vi "Main.vi"(11 "Module Admin":refnum<class "Delacor_lib_QMH_Module Admin.lvclass">) -> ()   [LabVIEW 2019, in "FunctionGenerator.lvlib"]
doc: "This template is based off of the Queued Message Handler design pattern and the Queued Message Handler project template that ships with LabVIEW.\n\nThe main difference is that the queue is private to this module and communication between modules is performed via Broadcast and Request events.\n\nRequest events are wrapped in public API methods and are handled in the Event Handling Loop (EHL) of this VI. Any module can register for Broadcast events sent by this module. The EHL generates messages based on user interface actions.\n\nThe Message Handling Loop (MHL) processes messages generated by the EHL, or by other messages. The messages are string values, so new messages can be added easily to the Message Cases case structure in the MHL. Each message cluster can also provide an optional value for Message Data, which is a variant that can be converted to whatever message-specific data is required.\n_____\nBased on DQMH Dev Tools: Project Template 7.1.0.1503."
uses:
  FunctionGenerator.lvlib
  <vilib>/Delacor/Delacor QMH/Libraries/Module Admin_class/Delacor_lib_QMH_Module Admin.lvclass
  Module Data--cluster.ctl
  Wake UP Continuous HL Argument--cluster.ctl
  <vilib>/Delacor/Delacor QMH/Libraries/Message Queue_class/Delacor_lib_QMH_Message Queue.lvclass/Delacor_lib_QMH_Message Queue.ctl
  Stop Argument--cluster.ctl
  <vilib>/Delacor/Delacor QMH/Libraries/Module Admin_class/Delacor_lib_QMH_Module Admin.lvclass/Delacor_lib_QMH_Module Admin.ctl
  Set Amplitude Argument--cluster.ctl
  Set Offset Argument--cluster.ctl
  Set Frecuency Argument--cluster.ctl
  Set Signal Type Argument--cluster.ctl
  Get Waveform Argument--cluster.ctl
  Get Waveform (Reply Payload)--cluster.ctl
  Start Continuous Acquisition Argument--cluster.ctl
  <vilib>/Utility/miscctls.llb/LVPointTypeDef.ctl
  <vilib>/Delacor/Delacor QMH/Libraries/Message Queue_class/Delacor_lib_QMH_Enqueue Message (Single).vi
  <vilib>/Delacor/Delacor QMH/Libraries/Module Admin_class/Delacor_lib_QMH_Get External Launch.vi
  <vilib>/Delacor/Delacor QMH/Libraries/Message Queue_class/Delacor_lib_QMH_Message Queue.lvclass
  <vilib>/measure/NI_MABase.lvlib
panel:
  out "error out":errorcluster
  out "Status":string
  in  "Simulate MHL Error":bool
  in  "Simulate EHL Error":bool
  # "Other processes communicate with this Module via its Public API (wrappers for its Request Events).\n\nThis Module communicates with other processes via its Broadcast Events.\nAny process that wants to receive these messages can register for this module's Broadcast events."
  # "This template is for the DQMH framework. See the block diagram for more information on how to use this template."
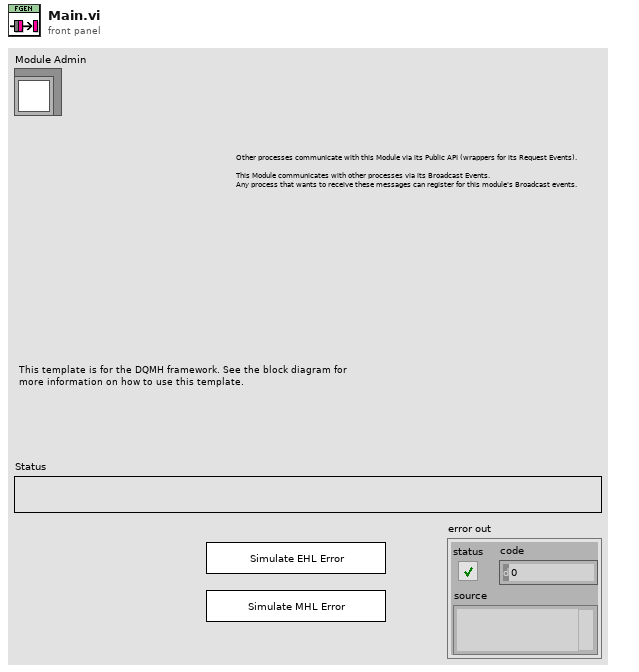
[diagram p1: front panel]
types:
  T1 = typedef "FunctionGenerator.lvlib/Request Events--cluster.ctl" = cluster{"Stop Module":refnum<user-event>, "Show Panel":refnum<user-event>, "Hide Panel":refnum<user-event>, "Get Module Execution Status":refnum<user-event>, "Show Diagram":refnum<user-event>, "Set Amplitude":refnum<user-event>, "Set Offset":refnum<user-event>, "Set Frecuency":refnum<user-event>, "Set Signal Type":refnum<user-event>, "Get Waveform":refnum<user-event>, "Private.Wake UP Continuous HL":refnum<user-event>, "Start Continuous Acquisition":refnum<user-event>, "Stop Continuous Generation":refnum<user-event>}
  T2 = typedef "FunctionGenerator.lvlib/Module Data--cluster.ctl" = cluster{"Status":string, "Amplitude":dbl, "Frecuency":dbl, "Offset":dbl, "signal type":enum16{"Sine Wave", "Triangle Wave", "Square Wave", "Sawtooth Wave"}}
  T3 = typedef "FunctionGenerator.lvlib/Wake UP Continuous HL Argument--cluster.ctl" = cluster{"Amplitude":dbl, "Frecuency":dbl, "Offset":dbl, "signal type":enum16{"Sine Wave", "Triangle Wave", "Square Wave", "Sawtooth Wave"}}
  T4 = enum32{"invalid lock state", "Not Locked", "Locked (No Password)", "Password-protected"}
  T5 = typedef "FunctionGenerator.lvlib/Stop Argument--cluster.ctl" = cluster{"Origin":string, "Exit via Stop Module Req?":bool, "Wait for Module to stop?":bool}
  T6 = typedef "FunctionGenerator.lvlib/Set Amplitude Argument--cluster.ctl" = cluster{"Amplitude":dbl}
  T7 = typedef "FunctionGenerator.lvlib/Set Offset Argument--cluster.ctl" = cluster{"Offset":dbl}
  T8 = typedef "FunctionGenerator.lvlib/Set Frecuency Argument--cluster.ctl" = cluster{"Frecuency":dbl}
  T9 = typedef "FunctionGenerator.lvlib/Set Signal Type Argument--cluster.ctl" = cluster{"signal type":enum16{"Sine Wave", "Triangle Wave", "Square Wave", "Sawtooth Wave"}}
  T10 = typedef "FunctionGenerator.lvlib/Get Waveform Argument--cluster.ctl" = cluster{"Wait Notifier":refnum<notifier>, "wait for reply":bool}
  T11 = typedef "FunctionGenerator.lvlib/Start Continuous Acquisition Argument--cluster.ctl" = cluster{"Boolean":bool}
  T12 = typedef "LVPointTypeDef.ctl" = cluster{"Horizontal":i16, "Vertical":i16}
  T13 = enum32{"Invalid", "Standard", "Closed", "Hidden", "Minimized", "Maximized"}
  T14 = typedef "FunctionGenerator.lvlib/Get Waveform (Reply Payload)--cluster.ctl" = cluster{"Waveform":waveform(dbl), "error":errorcluster}
  T15 = enum16{"Sine Wave", "Triangle Wave", "Square Wave", "Sawtooth Wave"}
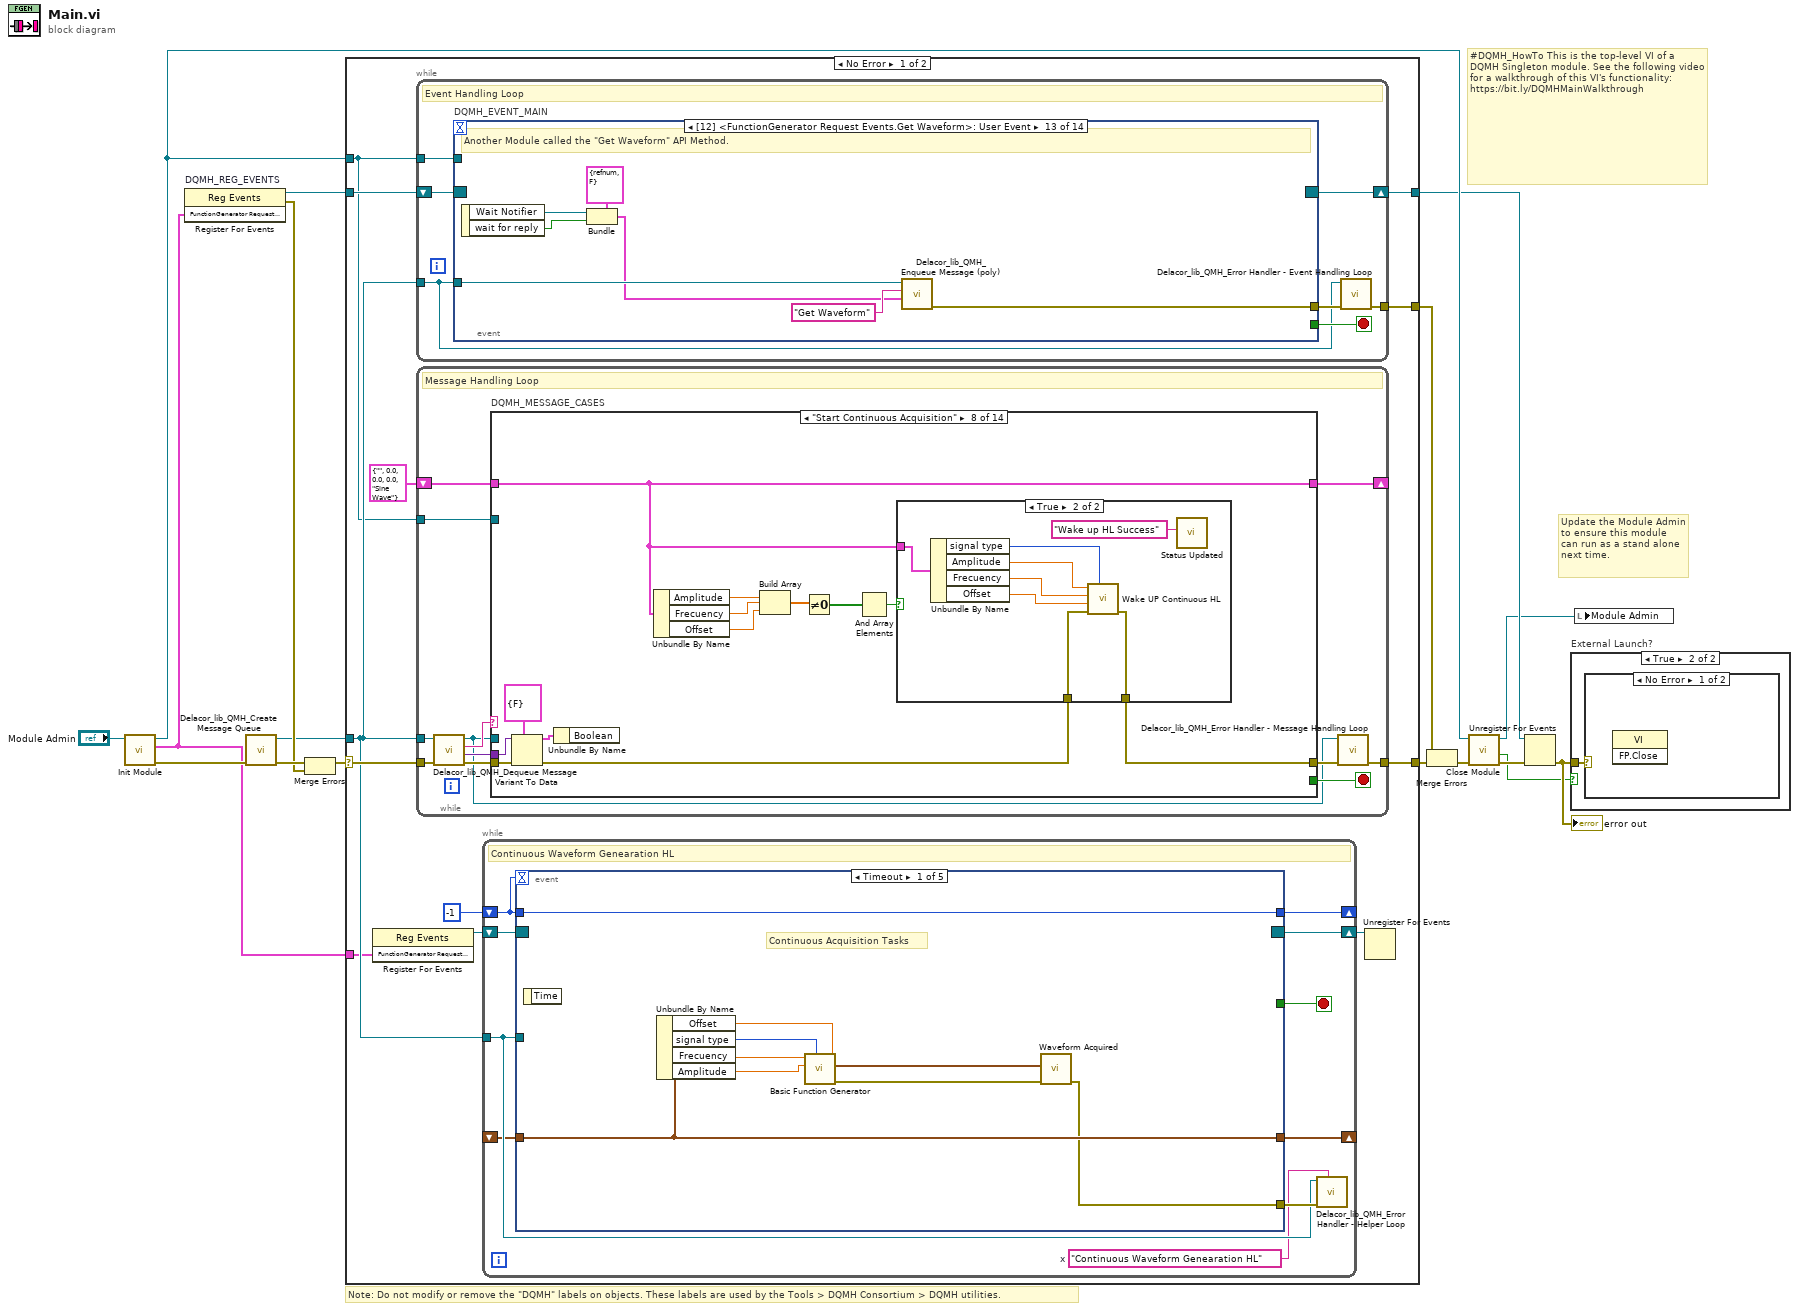
[diagram p0: block diagram]
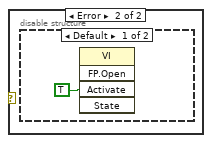
[diagram p3: hidden frame]
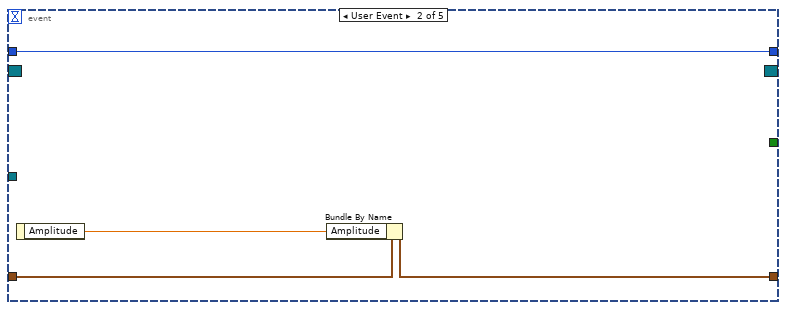
[diagram p5: hidden frame]
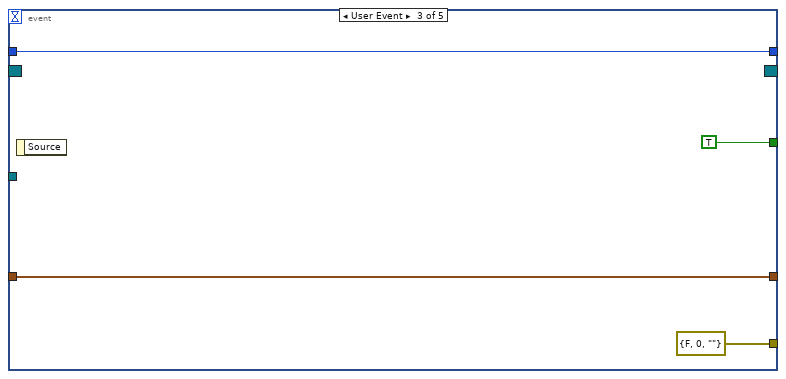
[diagram p6: hidden frame]
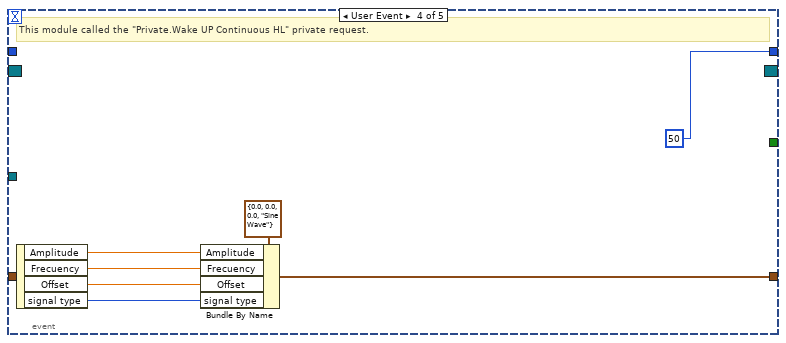
[diagram p7: hidden frame]
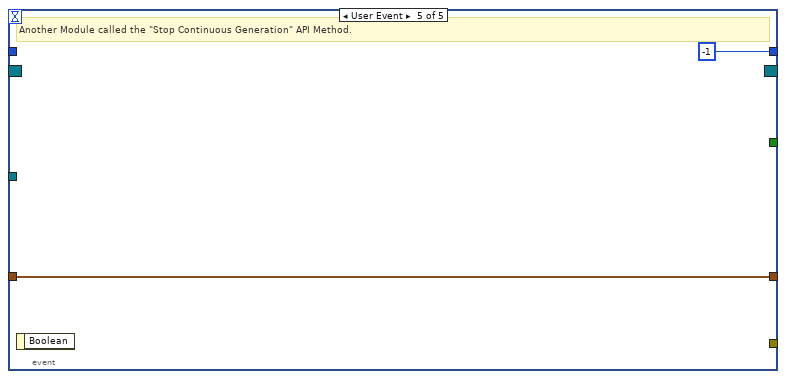
[diagram p8: hidden frame]
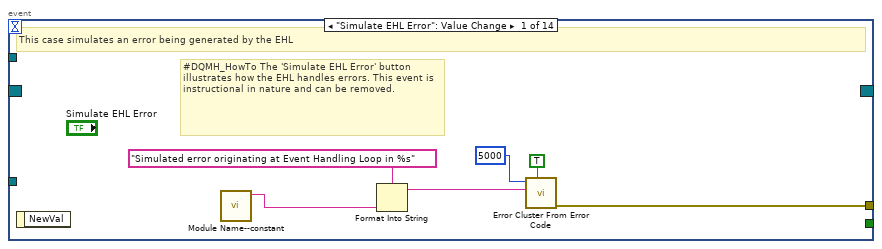
[diagram p9: hidden frame]
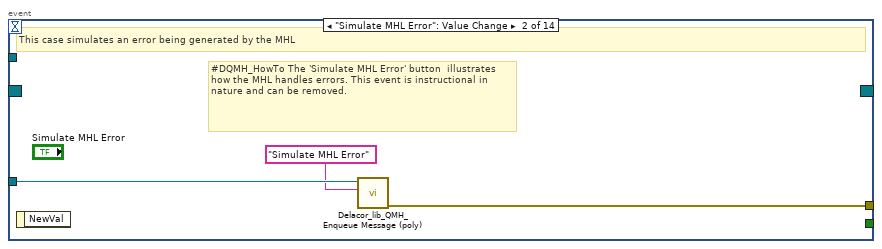
[diagram p10: hidden frame]
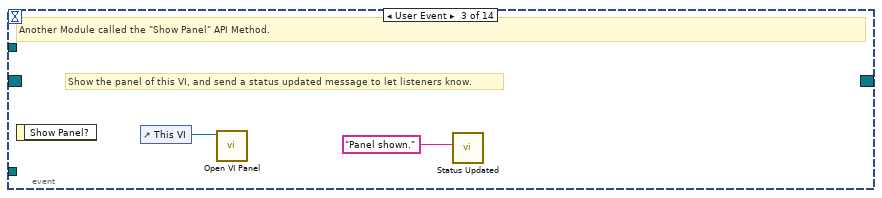
[diagram p11: hidden frame]
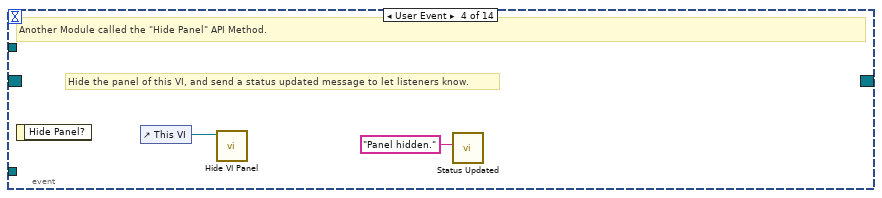
[diagram p12: hidden frame]
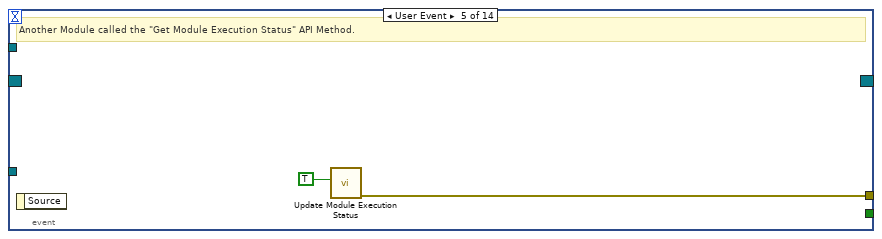
[diagram p13: hidden frame]
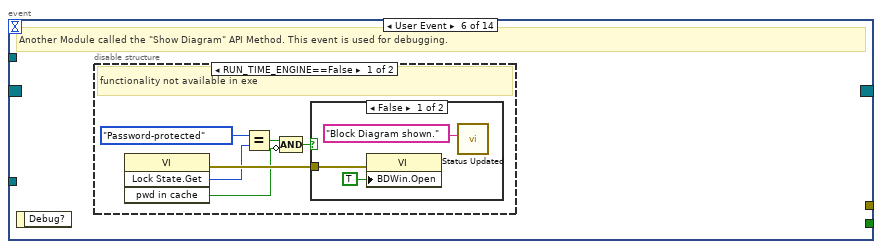
[diagram p14: hidden frame]
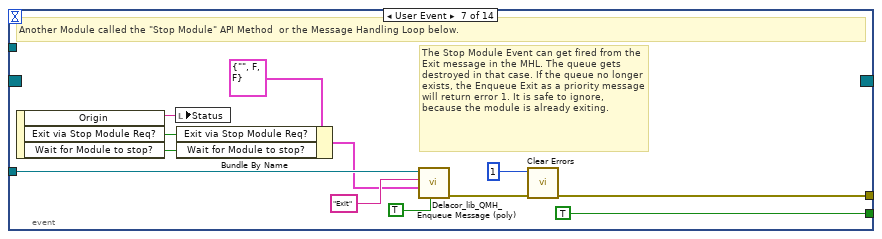
[diagram p17: hidden frame]
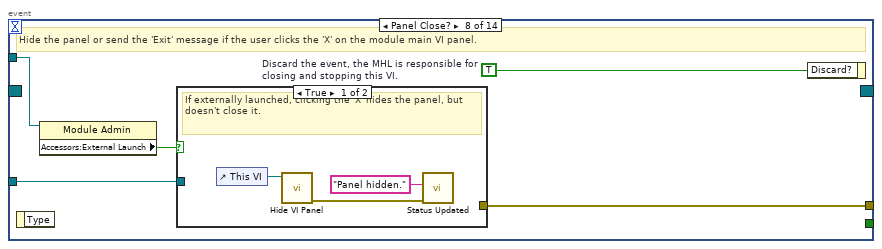
[diagram p18: hidden frame]
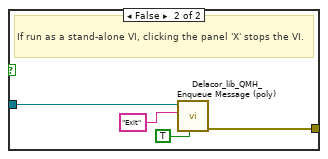
[diagram p19: hidden frame]
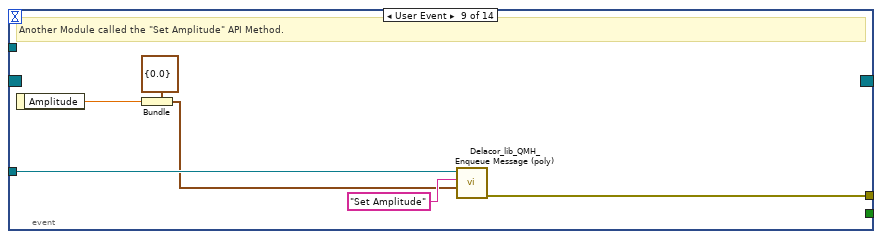
[diagram p20: hidden frame]
diagram:
  # "#DQMH_HowTo This is the top-level VI of a DQMH Singleton module. See the following video for a walkthrough of this VI's functionality: https://bit.ly/DQMHMainWalkthrough"
  # "Note: Do not modify or remove the \"DQMH\" labels on objects. These labels are used by the Tools > DQMH Consortium > DQMH utilities."
  # "Update the Module Admin to ensure this module can run as a stand alone next time."
  n1 = call "Init Module.vi"("Singleton Module Admin in"="Module Admin") -> ("error out"=w16:errorcluster, "FunctionGenerator Request Events"=w1:T1, "Singleton Module Admin out"=w8:refnum<class "Delacor_lib_QMH_Module Admin.lvclass">)  [unwired: 8 in]
  n2 = register-events "DQMH_REG_EVENTS"(w1) -> (reference out=w6:refnum<event-registration>, error out=w9:errorcluster)  [unwired: 2 in]
  n3 = call <vilib>:"Delacor_lib_QMH_Create Message Queue.vi"("error in"=w16) -> ("error out"=w11:errorcluster, "Message Queue"=w5:refnum<class "Delacor_lib_QMH_Message Queue.lvclass">)  [unwired: 9 in]
  n4 = Merge Errors(w11, w9) -> (w10:errorcluster)
  n5 = case shown="No Error" w10 {
    selector: w10 -> [w27 w336]
    tunnel: [w29 w335] -> w17
    tunnel: [w26 w334] -> w7
    tunnel: w6 -> [w24 w334]
    tunnel: w5 -> [w23 w329]
    tunnel: [w28 _] -> w14
    tunnel: w8 -> [w22 w330]
    tunnel: w1 -> [w21 _]
    frame No Error {
      n6 = register-events ("DQMH_HELPER_REGFOREVENTS")(w21) -> (reference out=w19:refnum<event-registration>)  [unwired: 2 in, 1 out]
      n7 = while {
        tunnel: w23 -> [w66]
        shift-right: [w69] -> w26
        shift-left: w24 -> [w70]
        tunnel: [w71] -> w28
        tunnel: w22 -> [w67]
        stop <- w68 stop-if-true
        # "Event Handling Loop"
        n8 = event "DQMH_EVENT_MAIN" shown="[12] <FunctionGenerator Request Events.Get Waveform>: User Event" {
          selector: w70 -> [_ _ _ _ _ _ _ _ _ _ _ _ _ _]
          dyn-events: [_ _ _ _ _ _ _ _ _ _ _ _ _ _] -> w69
          timeout: _ -> [_ _ _ _ _ _ _ _ _ _ _ _ _ _]
          tunnel: [_ _ _ _ _ _ TRUE ("Discard?") _ _ _ _ _ _ _] -> w68
          tunnel: w66 -> [_ w80 _ _ _ _ w104 w111 w125 w131 w137 w144 w151 w157]
          tunnel: [w78 w81 _ _ w87 _ w107 w113 w126 w132 w138 w139 w145 w152] -> w72
          tunnel: w67 -> [_ _ _ _ _ _ _ w110 _ _ _ _ _ _]
          event "Simulate EHL Error": Value Change {
            # "#DQMH_HowTo The 'Simulate EHL Error' button  illustrates how the EHL handles errors. This event is instructional in nature and can be removed."
            # "This case simulates an error being generated by the EHL"
            n9 = event-data() -> ()  [unwired: 1 in, 1 out]
            n10 = call "Module Name--constant.vi"() -> ("Module Name"=w75:string)  [unwired: 11 in]
            n11 = Format Into String(format string="Simulated error originating at Event Handling Loop in %s", w75) -> (resulting string=w76:string)  [unwired: 2 in, 1 out]
            n12 = call <vilib>:"Error Cluster From Error Code.vi"("show call chain? (False)"=TRUE, "error message (\"\")"=w76, "error code (0)"=5000) -> ("error out"=w78:errorcluster)  [unwired: 6 in]
          }
          event "Simulate MHL Error": Value Change {
            # "#DQMH_HowTo The 'Simulate MHL Error' button  illustrates how the MHL handles errors. This event is instructional in nature and can be removed."
            # "This case simulates an error being generated by the MHL"
            n13 = event-data() -> ()  [unwired: 1 in, 1 out]
            n14 = call-poly <vilib>:"Delacor_lib_QMH_Enqueue Message (poly).vi"("Message"="Simulate MHL Error", "Message Queue in"=w80) -> ("error out"=w81:errorcluster)  [unwired: 8 in, 1 out]
          }
          event User Event {
            # "Show the panel of this VI, and send a status updated message to let listeners know."
            # "Another Module called the \"Show Panel\" API Method."
            n15 = event-data() -> ()  [unwired: 1 in, 1 out]
            n16 = control-ref of="This VI"() -> (w83:refnum<vi>)
            n17 = call "Open VI Panel.vi"("VI"=w83) -> ()  [unwired: 10 in, 1 out]
            n18 = call "Status Updated.vi"("Status"="Panel shown." ("format string")) -> ()  [unwired: 10 in, 1 out]
          }
          event User Event {
            # "Hide the panel of this VI, and send a status updated message to let listeners know."
            # "Another Module called the \"Hide Panel\" API Method."
            n19 = event-data() -> ()  [unwired: 1 in, 1 out]
            n20 = control-ref of="This VI"() -> (w85:refnum<vi>)
            n21 = call "Hide VI Panel.vi"("VI"=w85) -> ()  [unwired: 10 in, 1 out]
            n22 = call "Status Updated.vi"("Status"="Panel hidden." ("format string")) -> ()  [unwired: 10 in, 1 out]
          }
          event User Event {
            # "Another Module called the \"Get Module Execution Status\" API Method."
            n23 = event-data() -> ()  [unwired: 1 in, 1 out]
            n24 = call "Update Module Execution Status.vi"("Running?"=TRUE) -> ("error out"=w87:errorcluster)  [unwired: 10 in]
          }
          event User Event {
            # "Another Module called the \"Show Diagram\" API Method. This event is used for debugging."
            n25 = event-data() -> ()  [unwired: 1 in, 1 out]
            n26 = disable-structure shown="RUN_TIME_ENGINE==False" {
              frame condition #0 (active) {
                # "functionality not available in exe"
                n27 = invoke on="Invoke Node" class="VI" method="Lock State.Get"() -> (error out=w93:errorcluster, "Get Lock State"=w92:T4, "pwd in cache"=w89:bool)  [unwired: 4 in, 1 out]
                n28 = Equal?(x=T4."Password-protected", y=w92) -> (x = y?=w90:bool)
                n29 = Compound Arithmetic op=AND(w90, invert w89) -> (w88:bool)
                n30 = case shown="False" w88 {
                  tunnel: w93 -> [w96 _]
                  frame False {
                    n31 = property on="Property Node" class="VI"(error in=w96, "BDWin.Open"=TRUE ("Block Diagram Window:Open")) -> ()  [unwired: 1 in, 2 out]
                    n32 = call "Status Updated.vi"("Status"="Block Diagram shown." ("format string")) -> ()  [unwired: 10 in, 1 out]
                  }
                  frame True {
                    # "Password-protected VI, and the password is not in the cache. Do not show the diagram."
                  }
                }
              }
              frame condition #1 {
              }
            }
          }
          event User Event {
            # "The Stop Module Event can get fired from the Exit message in the MHL. The queue gets destroyed in that case. If the queue no longer exists, the Enqueue Exit as a priority message will return error 1. It is safe to ignore, because the module is already exiting."
            # "Another Module called the \"Stop Module\" API Method  or the Message Handling Loop below."
            n33 = event-data() -> ("Origin"=w103:string, "Exit via Stop Module Req?"=w99:bool, "Wait for Module to stop?"=w98:bool)  [unwired: 1 in]
            n34 = local write "Status"(w103) -> ()
            n35 = Bundle By Name(cluster=T5 {"Origin"="", "Exit via Stop Module Req?"=FALSE, "Wait for Module to stop?"=FALSE} ("Stop Argument"), "Exit via Stop Module Req?"=w99, "Wait for Module to stop?"=w98) -> (w97:T5)
            n36 = call-poly <vilib>:"Delacor_lib_QMH_Enqueue Message (poly).vi"("Priority Message? (F)"=TRUE, "Message Data"=w97, "Message"="Exit", "Message Queue in"=w104) -> ("error out"=w108:errorcluster)  [unwired: 6 in, 1 out]
            n37 = call <vilib>:"Clear Errors.vi"("error in (no error)"=w108, "specific error code to clear (0: all)"=1) -> ("error out"=w107:errorcluster)  [unwired: 4 in, 1 out]
          }
          event Panel Close? {
            w112 = TRUE  # Discard the event, the MHL is responsible for closing and stopping this VI.
            # "Hide the panel or send the 'Exit' message if the user clicks the 'X' on the module main VI panel."
            n38 = event-data() -> ()  [unwired: 1 in, 1 out]
            n39 = property on="Property Node" class="Module Admin"(reference=w110) -> ("Accessors:External Launch"=w109:bool)  [unwired: 1 in, 2 out]
            n40 = case shown="True" w109 {
              tunnel: w111 -> [_ w119]
              tunnel: [_ w120] -> w113
              frame True {
                # "If externally launched, clicking the 'X' hides the panel, but doesn't close it."
                n41 = control-ref of="This VI"() -> (w115:refnum<vi>)
                n42 = call "Hide VI Panel.vi"("VI"=w115) -> ("error out"=w116:errorcluster)  [unwired: 10 in]
                n43 = call "Status Updated.vi"("error in"=w116, "Status"="Panel hidden." ("format string")) -> ()  [unwired: 9 in, 1 out]
              }
              frame False {
                # "If run as a stand-alone VI, clicking the panel 'X' stops the VI."
                n44 = call-poly <vilib>:"Delacor_lib_QMH_Enqueue Message (poly).vi"("Priority Message? (F)"=TRUE, "Message"="Exit", "Message Queue in"=w119) -> ("error out"=w120:errorcluster)  [unwired: 7 in, 1 out]
              }
            }
            n45 = event-data ("Event Filter Node")("Discard?"=w112) -> ()  [unwired: 1 in, 1 out]
          }
          event User Event {
            # "Another Module called the \"Set Amplitude\" API Method."
            n46 = event-data() -> ("Amplitude"=w121:dbl)  [unwired: 1 in]
            n47 = Bundle(cluster=T6 {"Amplitude"=0.0} ("Set Amplitude Argument"), "Amplitude"=w121) -> (w122:T6)
            n48 = call-poly <vilib>:"Delacor_lib_QMH_Enqueue Message (poly).vi"("Message Data"=w122, "Message"="Set Amplitude", "Message Queue in"=w125) -> ("error out"=w126:errorcluster)  [unwired: 7 in, 1 out]
          }
          event User Event {
            # "Another Module called the \"Set Offset\" API Method."
            n49 = event-data() -> ("Offset"=w127:dbl)  [unwired: 1 in]
            n50 = Bundle(cluster=T7 {"Offset"=0.0} ("Set Offset Argument"), "Offset"=w127) -> (w128:T7)
            n51 = call-poly <vilib>:"Delacor_lib_QMH_Enqueue Message (poly).vi"("Message Data"=w128, "Message"="Set Offset", "Message Queue in"=w131) -> ("error out"=w132:errorcluster)  [unwired: 7 in, 1 out]
          }
          event User Event {
            # "Another Module called the \"Set Frecuency\" API Method."
            n52 = event-data() -> ("Frecuency"=w133:dbl)  [unwired: 1 in]
            n53 = Bundle(cluster=T8 {"Frecuency"=0.0} ("Set Frecuency Argument"), "Frecuency"=w133) -> (w134:T8)
            n54 = call-poly <vilib>:"Delacor_lib_QMH_Enqueue Message (poly).vi"("Message Data"=w134, "Message"="Set Frecuency", "Message Queue in"=w137) -> ("error out"=w138:errorcluster)  [unwired: 7 in, 1 out]
          }
          event User Event {
            # "Another Module called the \"Set Signal Type\" API Method."
            n55 = event-data() -> ("signal type"=w140:T15)  [unwired: 1 in]
            n56 = Bundle(cluster=T9 {"signal type"=enum."Sine Wave"} ("Set Signal Type Argument"), "signal type"=w140) -> (w141:T9)
            n57 = call-poly <vilib>:"Delacor_lib_QMH_Enqueue Message (poly).vi"("Message Data"=w141, "Message"="Set Signal Type", "Message Queue in"=w144) -> ("error out"=w139:errorcluster)  [unwired: 7 in, 1 out]
          }
          event User Event {
            # "Another Module called the \"Get Waveform\" API Method."
            n58 = event-data() -> ("Wait Notifier"=w147:refnum<notifier>, "wait for reply"=w146:bool)  [unwired: 1 in]
            n59 = Bundle(cluster=T10 {"Wait Notifier"=refnum, "wait for reply"=FALSE} ("Get Waveform Argument"), "Wait Notifier"=w147, "wait for reply"=w146) -> (w148:T10)
            n60 = call-poly <vilib>:"Delacor_lib_QMH_Enqueue Message (poly).vi"("Message Data"=w148, "Message"="Get Waveform", "Message Queue in"=w151) -> ("error out"=w145:errorcluster)  [unwired: 7 in, 1 out]
          }
          event User Event {
            # "Another Module called the \"Start Continuous Acquisition\" API Method."
            n61 = event-data() -> ("Boolean"=w153:bool)  [unwired: 1 in]
            n62 = Bundle(cluster=T11 {"Boolean"=FALSE} ("Start Continuous Acquisition Argument"), "Boolean"=w153) -> (w154:T11)
            n63 = call-poly <vilib>:"Delacor_lib_QMH_Enqueue Message (poly).vi"("Message Data"=w154, "Message"="Start Continuous Acquisition", "Message Queue in"=w157) -> ("error out"=w152:errorcluster)  [unwired: 7 in, 1 out]
          }
        }
        n64 = call-dynamic "Delacor_lib_QMH_Error Handler - Event Handling Loop.vi"("error in"=w72, "Message Queue in"=w66) -> ("dup error in"=w71:errorcluster)  [unwired: 8 in, 1 out]
      }
      n65 = while {
        tunnel: w23 -> [w158]
        shift-right: [w164] -> _
        shift-left: T2 {"Status"="", "Amplitude"=0.0, "Frecuency"=0.0, "Offset"=0.0, "signal type"=enum."Sine Wave"} ("Data Cluster") -> [w165]
        tunnel: w27 -> [w169]
        tunnel: [w167] -> w29
        tunnel: w22 -> [w160]
        stop <- w163 stop-if-true
        # "Message Handling Loop"
        n66 = call-dynamic "Delacor_lib_QMH_Dequeue Message.vi"("error in"=w169, "Message Queue in"=w158) -> ("error out"=w168:errorcluster, "Message Data"=w161:variant, "Message"=w162:string, "Message Queue out"=w159:refnum<class "Delacor_lib_QMH_Message Queue.lvclass">)  [unwired: 6 in]
        n67 = case "DQMH_MESSAGE_CASES" shown="\"Start Continuous Acquisition\"" w162 {
          selector: w162 -> [_ _ _ _ _ _ _ _ _ _ _ _ _ w324]
          tunnel: w159 -> [_ _ _ _ _ _ _ _ _ _ _ w289 w312 _]
          tunnel: w168 -> [w187 w191 w201 w211 w221 w231 w248 w263 w275 w277 w286 w297 w318 w327]
          tunnel: [w185 w191 w200 w210 w220 w229 w239 w258 w274 w277 w285 w293 w313 w328] -> w166
          tunnel: w165 -> [w176 w190 w199 w209 w219 w230 w238 w251 w273 w276 w283 w291 w311 w325]
          tunnel: [w175 w190 w195 w205 w215 w225 w238 w251 w273 w276 w283 w291 w311 w325] -> w164
          tunnel: [_ _ _ _ _ _ _ _ _ _ _ _ w310 _] -> w163
          tunnel: w161 -> [_ _ w198 w208 w218 w228 w246 w262 _ _ _ w290 w309 _]
          tunnel: w160 -> [w177 _ _ _ _ _ _ _ _ _ _ w288 w304 _]
          frame "Initialize" {
            w171 = "Initial Message" ("Initial Message")
            # "#DQMH_CodeNeeded - Initialize the appearance of the front panel."
            # "#DQMH_CodeNeeded - Initialize your state data here."
            # "Initialize - Any operation that needs to be done before the module can receive messages. Synchronize Caller Events.vi will inform Start Module.vi that the module has launched and is ready to receive messages. Module Did Init.vi will broadcast that the module initialized."
            n68 = call "Synchronize Caller Events.vi"("error in"=w187, "Singleton Module Admin in"=w177) -> ("error out"=w186:errorcluster, "Singleton Module Admin out"=w172:refnum<class "Delacor_lib_QMH_Module Admin.lvclass">)  [unwired: 8 in]
            n69 = property on="Property Node" class="Module Admin"(reference=w172) -> ("Accessors:External Launch"=w181:bool)  [unwired: 1 in, 2 out]
            n70 = Select(t=T13."Hidden" ("State"), s=w181, f=T13."Standard" ("State")) -> (s? t:f=w178:T13)
            n71 = call "Module Name--constant.vi"() -> ("Module Name"=w184:string)  [unwired: 11 in]
            n72 = property on="Property Node" class="VI"("Front Panel.Title"=w184) -> (reference out=w183:refnum<vi>, error out=w189:errorcluster)  [unwired: 2 in]
            n73 = invoke on="Invoke Node" class="VI" method="FP.Open"(reference=w183, error in=w189, "State"=w178) -> (reference out=w182:refnum<vi>, error out=w188:errorcluster)  [unwired: 2 in, 3 out]
            n74 = Bundle By Name(cluster=w176, "Status"=w171) -> (w175:T2)
            n75 = invoke on="Invoke Node" class="VI" method="FP.Center"(reference=w182, error in=w188) -> ()  [unwired: 1 in, 3 out]
            n76 = property on="Pane" class="Pane"("Origin"=T12 {"Horizontal"=0, "Vertical"=0}) -> ()  [unwired: 2 in, 2 out]
            n77 = call "Module Name--constant.vi"() -> ("Module Name"=w173:string)  [unwired: 11 in]
            n78 = call "Module Did Init.vi"("error in"=w186, "Initialized?"=TRUE, "Origin"=w173) -> ("error out"=w185:errorcluster)  [unwired: 8 in]
            "Status" <- w171
          }
          frame "---Module Specific---" {
            # "Separator -- The following cases handle messages specific to this Module."
          }
          frame "Set Amplitude" {
            # "Set Amplitude"
            n79 = Variant To Data(error in=w201, type=T6 {"Amplitude"=0.0} ("Set Amplitude Argument"), Variant=w198) -> (data=w196:T6, error out=w200:errorcluster)
            n80 = Unbundle By Name(w196) -> ("Amplitude"=w193:dbl)
            n81 = Bundle By Name(cluster=w199, "Amplitude"=w193) -> (w195:T2)
            n82 = Format Into String(format string="Amplitude set to: %.2f", w193) -> (resulting string=w194:string)  [unwired: 2 in, 1 out]
            n83 = call "Status Updated.vi"("Status"=w194) -> ()  [unwired: 10 in, 1 out]
          }
          frame "Set Offset" {
            # "Set Offset"
            n84 = Variant To Data(error in=w211, type=T7 {"Offset"=0.0} ("Set Offset Argument"), Variant=w208) -> (data=w206:T7, error out=w210:errorcluster)
            n85 = Unbundle By Name(w206) -> ("Offset"=w202:dbl)
            n86 = Bundle By Name(cluster=w209, "Offset"=w202) -> (w205:T2)
            n87 = Format Into String(format string="Offset set to: %.2f", w202) -> (resulting string=w204:string)  [unwired: 2 in, 1 out]
            n88 = call "Status Updated.vi"("Status"=w204) -> ()  [unwired: 10 in, 1 out]
          }
          frame "Set Frecuency" {
            # "Set Frecuency"
            n89 = Variant To Data(error in=w221, type=T8 {"Frecuency"=0.0} ("Set Frecuency Argument"), Variant=w218) -> (data=w216:T8, error out=w220:errorcluster)
            n90 = Unbundle By Name(w216) -> ("Frecuency"=w212:dbl)
            n91 = Bundle By Name(cluster=w219, "Frecuency"=w212) -> (w215:T2)
            n92 = Format Into String(format string="Frecuency set to: %.2f", w212) -> (resulting string=w214:string)  [unwired: 2 in, 1 out]
            n93 = call "Status Updated.vi"("Status"=w214) -> ()  [unwired: 10 in, 1 out]
          }
          frame "Set Signal Type" {
            # "Set Signal Type"
            n94 = Variant To Data(error in=w231, type=T9 {"signal type"=enum."Sine Wave"} ("Set Signal Type Argument"), Variant=w228) -> (data=w226:T9, error out=w229:errorcluster)
            n95 = Unbundle By Name(w226) -> ("signal type"=w222:T15)
            n96 = Bundle By Name(cluster=w230, "signal type"=w222) -> (w225:T2)
            n97 = Format Into String(format string="Signal type set to: %s", w222) -> (resulting string=w224:string)  [unwired: 2 in, 1 out]
            n98 = call "Status Updated.vi"("Status"=w224) -> ()  [unwired: 10 in, 1 out]
          }
          frame "Get Waveform" {
            # "Get waveform"
            n99 = Variant To Data(error in=w248, type=T10 {"Wait Notifier"=refnum, "wait for reply"=FALSE} ("Get Waveform Argument"), Variant=w246) -> (data=w244:T10, error out=w247:errorcluster)
            n100 = Unbundle By Name(w244) -> ("Wait Notifier"=w243:refnum<notifier>, "wait for reply"=w242:bool)
            n101 = Unbundle By Name(w238) -> ("Offset"=w236:dbl, "signal type"=w237:T15, "Frecuency"=w235:dbl, "Amplitude"=w234:dbl)
            n102 = call <vilib>:"Basic Function Generator.vi"("offset"=w236, "signal type"=w237, "amplitude"=w234, "frequency"=w235) -> ("error out"=w232:errorcluster, "signal out"=w233:waveform(dbl))  [unwired: 5 in, 1 out]
            n103 = call "Waveform Acquired.vi"("error in"=w232, "Waveform"=w233) -> ()  [unwired: 9 in, 1 out]
            n104 = Bundle By Name(cluster=T14 {"Waveform"={"t0"=timestamp(0 s since 1904-01-01), "dt"=1.0, "Y"=[]}, "error"={"status"=FALSE, "code"=0, "source"=""}} ("Get Waveform (Reply Payload)"), "Waveform"=w233, "error"=w232) -> (w241:T14)
            n105 = Merge Errors(w247, w232) -> (w239:errorcluster)
            n106 = case "DQMH_FIRE_NOTIFIER" shown="True" w242 {
              tunnel: w243 -> [_ w250]
              tunnel: w241 -> [_ w249]
              frame False {
              }
              frame True {
                n107 = Send Notification(notification=w249, notifier=w250) -> ()  [unwired: 1 in, 2 out]
              }
            }
          }
          frame "Start Continuous Acquisition" {
            n108 = Variant To Data(error in=w263, type=T11 {"Boolean"=FALSE} ("Start Continuous Acquisition Argument"), Variant=w262) -> (data=w260:T11, error out=w259:errorcluster)
            n109 = Unbundle By Name(w260) -> ()  [unwired: 1 out]
            n110 = Unbundle By Name(w251) -> ("Amplitude"=w257:dbl, "Frecuency"=w256:dbl, "Offset"=w255:dbl)
            n111 = Build Array(w257, w256, w255) -> (w254:dbl[])
            n112 = Not Equal To 0?(x=w254) -> (x != 0?=w253:bool[])
            n113 = And Array Elements(Boolean array=w253) -> (logical AND=w252:bool)
            n114 = case shown="True" w252 {
              tunnel: w259 -> [w264 w272]
              tunnel: [w264 w271] -> w258
              tunnel: w251 -> [_ w269]
              frame False {
              }
              frame True {
                n115 = Unbundle By Name(w269) -> ("signal type"=w268:T15, "Amplitude"=w267:dbl, "Frecuency"=w266:dbl, "Offset"=w265:dbl)
                n116 = call "Wake UP Continuous HL.vi"("signal type"=w268, "error in"=w272, "Offset"=w265, "Frecuency"=w266, "Amplitude"=w267) -> ("error out"=w271:errorcluster)  [unwired: 6 in]
                n117 = call "Status Updated.vi"("Status"="Wake up HL Success") -> ()  [unwired: 10 in, 1 out]
              }
            }
          }
          frame "---Copy This Frame---" {
            # "Duplicate this frame when creating new messages.  Change this comment in the duplicated frame to describe this message."
            n118 = Merge Errors(w275) -> (w274:errorcluster)
          }
          frame "---Exit and Error Handling---" {
            # "Separator - The following cases handle errors and exit messages."
          }
          frame "Simulate MHL Error" {
            # "#DQMH_HowTo The 'Simulate MHL Error' button  illustrates how the MHL handles errors. This event is instructional in nature and can be removed."
            # "Simulate an error occurring at the MHL"
            n119 = call "Module Name--constant.vi"() -> ("Module Name"=w279:string)  [unwired: 11 in]
            n120 = Format Into String(format string="Simulated error originating at Message Handling Loop in %s", w279) -> (resulting string=w280:string)  [unwired: 2 in, 1 out]
            n121 = call <vilib>:"Error Cluster From Error Code.vi"("show call chain? (False)"=TRUE, "error message (\"\")"=w280, "error code (0)"=5001) -> ("error out"=w284:errorcluster)  [unwired: 6 in]
            n122 = Merge Errors(w286, w284) -> (w285:errorcluster)
          }
          frame "Error" {
            # "#DQMH_CodeRecommended - If the module is running in standalone mode (External Launch = FALSE), this code will pop up an error dialog and call the 'Exit' message if an error occurs. Add more fine-grained error management here."
            # "Error - Check the error message data and respond accordingly. This message is sent by the \"Error Handler\" VIs at the end of each loop in this application."
            n123 = property on="Property Node" class="Module Admin"(reference=w288) -> ("Accessors:External Launch"=w287:bool)  [unwired: 1 in, 2 out]
            n124 = Variant To Data(error in=w297, type=errorcluster {"status"=FALSE, "code"=0, "source"=""} ("error constant"), Variant=w290) -> (data=w292:errorcluster, error out=w295:errorcluster)
            n125 = local write "error out"(w292) -> ()
            n126 = call "Error Reported.vi"("Error"=w292) -> ()  [unwired: 10 in, 1 out]
            n127 = case shown="False" w287 {
              tunnel: [w302 _] -> w294
              tunnel: w289 -> [w300 _]
              tunnel: w292 -> [w301 _]
              frame False {
                n128 = disable-structure shown="Default" {
                  disable-tunnel: w301 -> [w303 _]
                  frame condition #0 (active) {
                    # "If the module is running standalone, then pop up an error dialog and call the \"Exit\" message."
                    n129 = call <vilib>:"Simple Error Handler.vi"("error in (no error)"=w303) -> ()  [unwired: 4 in, 5 out]
                  }
                  frame condition #1 {
                    # "To prevent the Simple Error Handler VI from being loaded (e.g. when deploying to a Real-Time target), add the Conditional Disable Symbol \"DQMH_Disable_SEH\" to your project and set it to TRUE."
                  }
                }
                n130 = call-poly <vilib>:"Delacor_lib_QMH_Enqueue Message (poly).vi"("Priority Message? (F)"=TRUE, "Message"="Exit", "Message Queue in"=w300) -> ("error out"=w302:errorcluster)  [unwired: 7 in, 1 out]
              }
              frame True {
                # "If the module was launched externally, calling the Error Reported broadcast VI is the only action performed by the \"Error\" message. The module's caller can then process the error appropriately."
              }
            }
            n131 = Merge Errors(w295, w294) -> (w293:errorcluster)
          }
          frame "Exit" {
            w308 = 91  # 91: not all Exit messages will have an argument
            w310 = TRUE  # Stop the VI
            # "Release the message queue reference"
            # "#DQMH_CodeNeeded - Add any required cleanup code here."
            # "Exit - Exit the application."
            n132 = Variant To Data(error in=w318, type=T5 {"Origin"="", "Exit via Stop Module Req?"=FALSE, "Wait for Module to stop?"=FALSE} ("Stop Argument"), Variant=w309) -> (data=w306:T5, error out=w315:errorcluster)
            n133 = call <vilib>:"Clear Errors.vi"("error in (no error)"=w315, "specific error code to clear (0: all)"=w308) -> ("error out"=w317:errorcluster)  [unwired: 4 in, 1 out]
            n134 = control-ref of="This VI"() -> (w305:refnum<vi>)
            n135 = call-dynamic "Delacor_lib_QMH_Release Message Queue.vi"("error in"=w317, "Message Queue"=w312) -> ("error out"=w316:errorcluster)  [unwired: 9 in]
            n136 = call "Handle Exit.vi"("Stop Argument"=w306, "Admin in"=w304, "VI reference"=w305) -> ("error out"=w314:errorcluster)  [unwired: 7 in, 1 out]
            n137 = Merge Errors(w316, w314) -> (w313:errorcluster)
            n138 = call "Error Reported.vi"("Error"=w313) -> ()  [unwired: 10 in, 1 out]
          }
          frame Default {
            # "'Default' case only runs if there is a message that isn't defined in any of the other cases.  Output a programming error."
            n139 = call "Module Name--constant.vi"() -> ("Module Name"=w323:string)  [unwired: 11 in]
            n140 = Format Into String(format string="The invalid message string \"%s\" was received in the Message Handling Loop for module \"%s\".", w324, w323) -> (resulting string=w319:string)  [unwired: 2 in, 1 out]
            n141 = call <vilib>:"Error Cluster From Error Code.vi"("show call chain? (False)"=TRUE, "error message (\"\")"=w319, "error code (0)"=1) -> ("error out"=w326:errorcluster)  [unwired: 6 in]
            n142 = Merge Errors(w327, w326) -> (w328:errorcluster)
          }
        }
        n143 = call-dynamic "Delacor_lib_QMH_Error Handler - Message Handling Loop.vi"("error in"=w166, "Message Queue in"=w159) -> ("dup error in"=w167:errorcluster)  [unwired: 8 in, 1 out]
      }
      n144 = while "DQMH_HELPER_LOOP" {
        shift-right: [w39] -> _
        shift-left: -1 -> [w38]
        shift-right: [w36] -> w20
        shift-left: w19 -> [w37]
        tunnel: w23 -> [w33]
        shift-right: [w31] -> _
        shift-left: _ -> [w30]
        stop <- w35 stop-if-true
        w32 = "Continuous Waveform Genearation HL"  # x
        # "Continuous Waveform Genearation HL"
        n145 = event "DQMH_HELPER_EVENT_STRUCTURE" shown="[0] Timeout" {
          selector: w37 -> [_ _ _ _ _]
          dyn-events: [_ _ _ _ _] -> w36
          timeout: w38 -> [_ _ _ _ _]
          tunnel: w38 -> [w48 w52 w56 _ _]
          tunnel: [w48 w52 w56 50 -1] -> w39
          tunnel: [_ _ TRUE _ _] -> w35
          tunnel: [w44 _ errorcluster {"status"=FALSE, "code"=0, "source"=""} ("error constant") _ _] -> w34
          tunnel: w33 -> [_ _ _ _ _]
          tunnel: [w47 w50 w53 w58 w65] -> w31
          tunnel: w30 -> [w47 w51 w53 _ w65]
          event Timeout {
            # "Continuous Acquisition Tasks"
            n146 = event-data() -> ()  [unwired: 1 in, 1 out]
            n147 = Unbundle By Name(w47) -> ("Offset"=w42:dbl, "signal type"=w43:T15, "Frecuency"=w41:dbl, "Amplitude"=w40:dbl)
            n148 = call <vilib>:"Basic Function Generator.vi"("offset"=w42, "signal type"=w43, "amplitude"=w40, "frequency"=w41) -> ("error out"=w45:errorcluster, "signal out"=w46:waveform(dbl))  [unwired: 5 in, 1 out]
            n149 = call "Waveform Acquired.vi"("error in"=w45, "Waveform"=w46) -> ("error out"=w44:errorcluster)  [unwired: 9 in]
          }
          event User Event {
            n150 = event-data() -> ("Amplitude"=w49:dbl)  [unwired: 1 in]
            n151 = Bundle By Name(cluster=w51, "Amplitude"=w49) -> (w50:T3)
          }
          event User Event {
            n152 = event-data() -> ()  [unwired: 1 in, 1 out]
          }
          event User Event {
            # "This module called the \"Private.Wake UP Continuous HL\" private request."
            n153 = event-data() -> ("Amplitude"=w62:dbl, "Frecuency"=w59:dbl, "Offset"=w60:dbl, "signal type"=w61:T15)  [unwired: 1 in]
            n154 = Bundle By Name(cluster=T3 {"Amplitude"=0.0, "Frecuency"=0.0, "Offset"=0.0, "signal type"=enum."Sine Wave"}, "Amplitude"=w62, "Frecuency"=w59, "Offset"=w60, "signal type"=w61) -> (w58:T3)
          }
          event User Event {
            # "Another Module called the \"Stop Continuous Generation\" API Method."
            n155 = event-data() -> ()  [unwired: 1 in, 1 out]
          }
        }
        n156 = call-dynamic "Delacor_lib_QMH_Error Handler - Helper Loop.vi"("Error Debug"=w32, "error in"=w34, "Message Queue in"=w33) -> ()  [unwired: 7 in, 2 out]
      }
      n157 = Unregister For Events(event registration refnum=w20) -> ()  [unwired: 1 in, 1 out]
    }
    frame Error {
      # "Synchronize Caller Events.vi will inform Start Module.vi that the module has launched and will let the code calling Start Module.vi register for broadcasts and would permit the caller receive the broadcast that an error occurred at launch time."
      n158 = call-dynamic "Delacor_lib_QMH_Release Message Queue.vi"("error in"=w336, "Message Queue"=w329) -> ("error out"=w335:errorcluster)  [unwired: 9 in]
      n159 = call "Synchronize Caller Events.vi"("Singleton Module Admin in"=w330) -> ("error out"=w337:errorcluster)  [unwired: 9 in, 1 out]
      n160 = call "Module Name--constant.vi"() -> ("Module Name"=w333:string)  [unwired: 11 in]
      n161 = Format Into String(format string="An error occurred during initialization. %s is no longer running.", w333) -> (resulting string=w331:string)  [unwired: 2 in, 1 out]
      n162 = Merge Errors(w335, w337) -> (w338:errorcluster)
      n163 = call "Error Reported.vi"("Additional Information"=w331, "Error"=w338) -> ()  [unwired: 9 in, 1 out]
    }
  }
  n164 = Merge Errors(w14, w17) -> (w13:errorcluster)
  n165 = call "Close Module.vi"("error in"=w13, "Module Admin in"=w8) -> ("error out"=w15:errorcluster, "External Launch"=w2:bool, "Module Admin out"=w3:refnum<class "Delacor_lib_QMH_Module Admin.lvclass">)  [unwired: 7 in]
  n166 = Unregister For Events(event registration refnum=w7, error in=w15) -> (error out=w12:errorcluster)
  "error out" <- w12
  n167 = case "External Launch?" shown="True" w2 {
    tunnel: w12 -> [_ w339]
    frame False {
    }
    frame True {
      n168 = case shown="No Error" w339 {
        frame No Error {
          n169 = invoke on="Invoke Node" class="VI" method="FP.Close"() -> ()  [unwired: 3 in, 3 out]
        }
        frame Error {
          n170 = disable-structure shown="Default" {
            frame condition #0 (active) {
              n171 = invoke class="VI" method="FP.Open"("Activate"=TRUE ("Activate?")) -> ()  [unwired: 4 in, 5 out]
            }
            frame condition #1 {
              # "Don't show panel on error if running inside a built EXE."
            }
          }
        }
      }
    }
  }
  n172 = local write "Module Admin"(w3) -> ()
